vi "VS_CheckStimState.vi"(0 "Engine Reference(in)":refnum<k7>, 1 "Condition Run?":bool, 5 "Sequence File Ref(in)":refnum<k7>, 7 "VeriStand version info":T1, 11 "error in":errorcluster, 12 "Step Group":i32(ring) items=["StepGroup_Setup", "StepGroup_Main", "StepGroup_Cleanup"], 13 "Step Index":i32) -> (4 "Engine reference(out)":refnum<k7>, 6 "Sequence File Ref(out)":refnum<k7>, 8 "VeriStand version info (out)":T1, 15 "error out":errorcluster)   [LabVIEW 2010]
doc: "This VI creates a TestStand step that check for the Stimulus Profile Manager state."
uses:
  Ctls/dotNetAssemblyInfo.ctl
  Ctls/VSModuleTokens.ctl
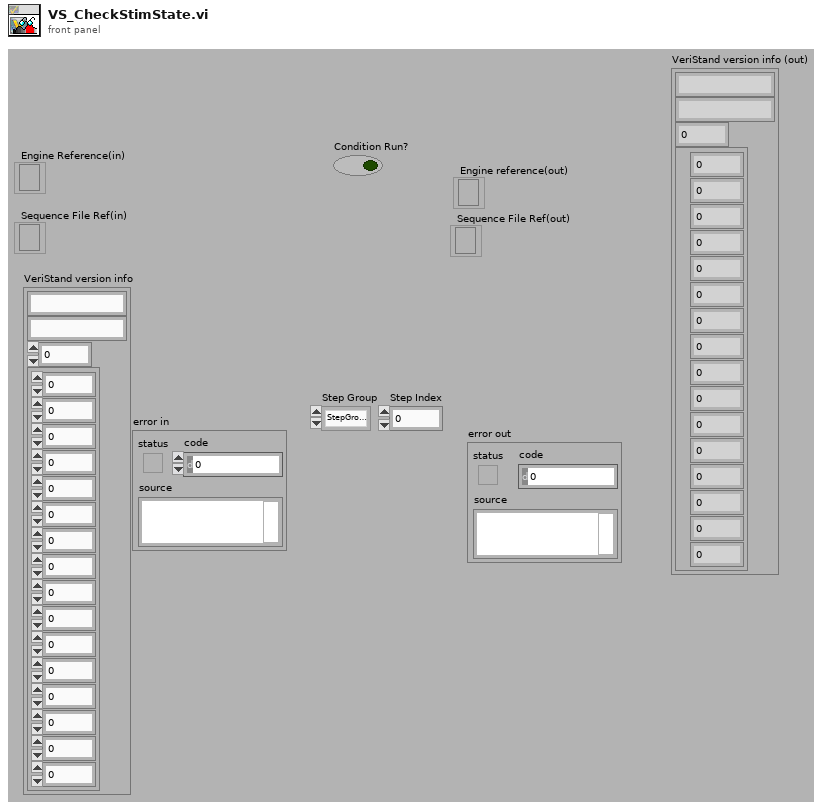
[diagram p1: front panel]
types:
  T1 = typedef "dotNetAssemblyInfo.ctl" = cluster{"VeriStand.exe Path":string, "Assembly":string, "Constructor Token":i32, "Module Token":T2}
  T2 = typedef "VSModuleTokens.ctl" = cluster{"GetIWorkspaceToken":i32, "GetIStimulusToken":i32, "GetIModelManagerToken":i32, "GetIProjectToken":i32, "RunProjectToken":i32, "CloseProjectToken":i32, "RunWorkspaceToken":i32, "StopWorkspaceToken":i32, "SetSingleChannelToken":i32, "SetMultipleParametersToken":i32, "RunStimulusToken":i32, "GetStimulusStateToken":i32, "Open WorkspaceToken":i32, "DeployToken":i32, "UndeployToken":i32, "QuitToken":i32}
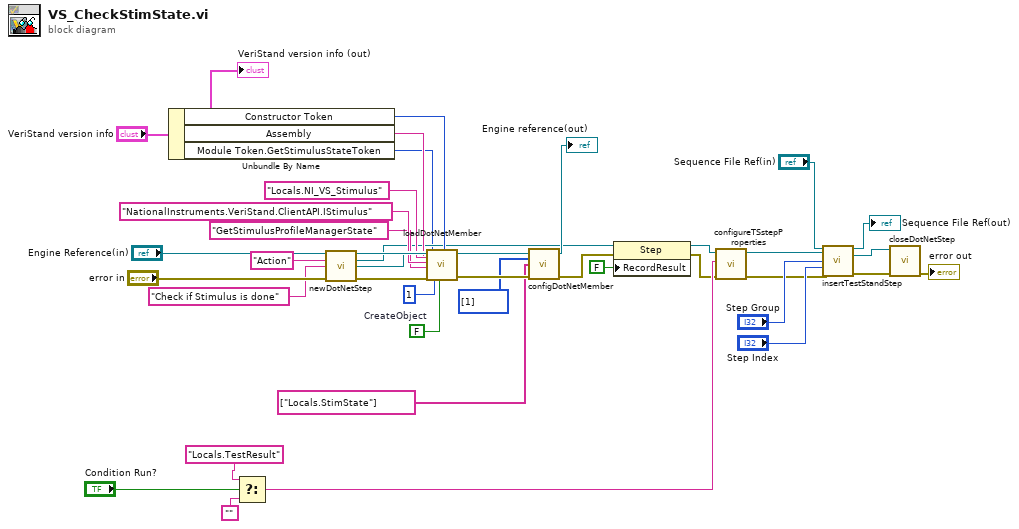
[diagram p0: block diagram]
diagram:
  w22 = FALSE  # CreateObject
  n1 = Unbundle By Name("VeriStand version info") -> ("Constructor Token"=w16:i32, "Assembly"=w17:string, "Module Token.GetStimulusStateToken"=w6:i32)
  n2 = Select(t="Locals.TestResult", s="Condition Run?", f="") -> (s? t:f=w8:string)
  n3 = call "newDotNetStep.vi"("Engine reference"="Engine Reference(in)", "stepType"="Action", "Step Name"="Check if Stimulus is done", "error in"="error in") -> ("Engine reference(out)"=→"Engine reference(out)":refnum<k7>, "NewStep (out)"=w10:refnum<k7>, "dotNetModule(out)"=w26:refnum<k7>, "error out"=w38:errorcluster)  [unwired: 8 in]
  n4 = call "loadDotNetMember.vi"("dotNetModule"=w26, "Strong Assembly path"=w17, "ClassName"="NationalInstruments.VeriStand.ClientAPI.IStimulus", "MemberName"="GetStimulusProfileManagerState", "Member token"=w6, "error in(no error)"=w38, "ClassReference"="Locals.NI_VS_Stimulus", "Call Member?"=1 ("Call Memeber?"), "CreateObject"=w22, "Constructor Token"=w16) -> ("dotNetModule(out)"=w21:refnum<k7>, "error out"=w20:errorcluster)  [unwired: 8 in]
  n5 = call "configDotNetMember.vi"("dotNetModule"=w21, "Index array"=i32[] [1], "Parameter Value array"=string[] ["Locals.StimState"], "error in (no error)"=w20) -> ("error out"=w3:errorcluster)  [unwired: 11 in]
  n6 = property class="Step"(reference=w10, error in=w3, "RecordResult"=FALSE) -> (reference out=w4:refnum<k7>, error out=w2:errorcluster)
  n7 = call "configureTSstepProperties.vi"("error in"=w2, "Precondition"=w8, "NewStep (in)"=w4) -> ("error out"=w7:errorcluster, "NewStep (out)"=w9:refnum<k7>)  [unwired: 7 in]
  n8 = call "insertTestStandStep.vi"("Sequence File Ref"="Sequence File Ref(in)", "Step to insert"=w9, "Step Group"="Step Group", "index"="Step Index", "error out"=w7) -> ("Sequence File Ref(out)"=→"Sequence File Ref(out)":refnum<k7>, "Step to insert (out)"=w37:refnum<k7>, "error out"=w35:errorcluster)  [unwired: 8 in]
  n9 = call "closeDotNetStep.vi"("error in"=w35, "NewStep"=w37) -> ("error out"=→"error out":errorcluster)  [unwired: 9 in]
  "VeriStand version info (out)" <- "VeriStand version info"
